vi "SetupROI.vi"(8 "error in (no error)":errorcluster, 10 "keep_first":u8) -> (0 "error out":errorcluster)   [LabVIEW 2015, in "ESLSCDLL.lvlib"]
uses:
  ESLSCDLL.lvlib
  Globals.vi
panel:
  # "if 0 every odd region is shown\nif 1 every even region is shown"
  # "number of regions 2...8"
  # "lines in camera"
  # "number of lines for each region.\nWhen selection 0 for the first region,\nthe lines are equally distributed over all regions.\nThe sum of all regions should equal lines."
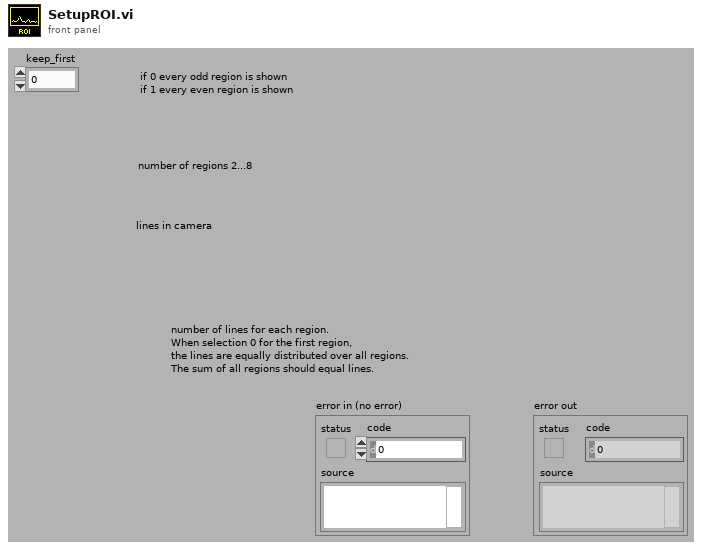
[diagram p1: front panel]
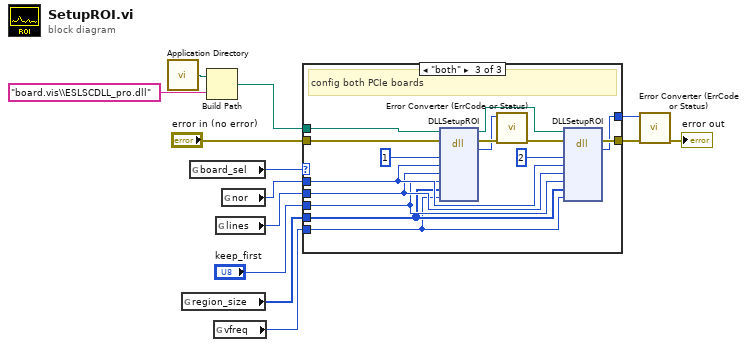
[diagram p0: block diagram]
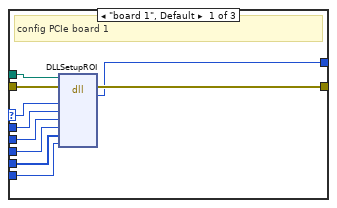
[diagram p2: hidden frame]
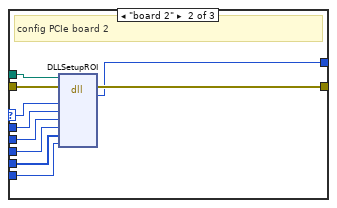
[diagram p3: hidden frame]
diagram:
  n1 = call <vilib>:"Application Directory.vi"() -> ("Application Directory"=w3:path)
  n2 = global read "Globals.vi" "region_size"() -> (w8:u32[])
  n3 = global read "Globals.vi" "board_sel"() -> (w7:enum32{"0", "board 1", "board 2", "both"})
  n4 = Build Path(base path=w3, name or relative path="board.vis\\ESLSCDLL_pro.dll") -> (appended path=w1:path)
  n5 = global read "Globals.vi" "vfreq"() -> (w4:u32)
  n6 = global read "Globals.vi" "lines"() -> (w5:u32)
  n7 = global read "Globals.vi" "nor"() -> (w6:u32)
  n8 = case shown="\"both\"" w7 {
    selector: w7 -> [w23 w33 _]
    tunnel: w6 -> [w22 w32 w46]
    tunnel: w5 -> [w21 w31 w45]
    tunnel: "keep_first" -> [w20 w30 w44]
    tunnel: w8 -> [w19 w29 w43]
    tunnel: w4 -> [w18 w28 w42]
    tunnel: "error in (no error)" -> [w17 w25 w41]
    tunnel: [w16 w27 w37] -> w10
    tunnel: [w15 w26 w36] -> w9
    tunnel: w1 -> [w14 w24 w35]
    frame "board 1", Default {
      # "config PCIe board 1"
      n9 = dll-call lib="C:/ENTW/PCIE/LV64/board.vis/ESLSCDLL_pro.dll" fn="DLLSetupROI" ("lwlscdll.dll:DLLRsTOREG")(path in=w14, error in=w17, "drv"=w23, "number_of_regions"=w22, "lines"=w21, "keep_first"=w20, "region_size"=w19, "vfreq"=w18) -> (error out=w16:errorcluster, "es_status_codes"=w15:i32)  [unwired: 7 in, 1 out]
    }
    frame "board 2" {
      # "config PCIe board 2"
      n10 = dll-call lib="C:/ENTW/PCIE/LV64/board.vis/ESLSCDLL_pro.dll" fn="DLLSetupROI" ("lwlscdll.dll:DLLRsTOREG")(path in=w24, error in=w25, "drv"=w33, "number_of_regions"=w32, "lines"=w31, "keep_first"=w30, "region_size"=w29, "vfreq"=w28) -> (error out=w27:errorcluster, "es_status_codes"=w26:i32)  [unwired: 7 in, 1 out]
    }
    frame "both" {
      # "config both PCIe boards"
      n11 = dll-call lib="C:/ENTW/PCIE/LV64/board.vis/ESLSCDLL_pro.dll" fn="DLLSetupROI" ("lwlscdll.dll:DLLRsTOREG")(path in=w35, error in=w41, "drv"=u32 1, "number_of_regions"=w46, "lines"=w45, "keep_first"=w44, "region_size"=w43, "vfreq"=w42) -> (path out=w34:path, error out=w40:errorcluster, "es_status_codes"=w39:i32)  [unwired: 7 in]
      n12 = call "Error Converter (ErrCode or Status).vi"("error in (no error)"=w40, "error code"=w39) -> ("error out"=w38:errorcluster)  [unwired: 9 in]
      n13 = dll-call lib="C:/ENTW/PCIE/LV64/board.vis/ESLSCDLL_pro.dll" fn="DLLSetupROI" ("lwlscdll.dll:DLLRsTOREG")(path in=w34, error in=w38, "drv"=u32 2, "number_of_regions"=w46, "lines"=w45, "keep_first"=w44, "region_size"=w43, "vfreq"=w42) -> (error out=w37:errorcluster, "es_status_codes"=w36:i32)  [unwired: 7 in, 1 out]
    }
  }
  n14 = call "Error Converter (ErrCode or Status).vi"("error in (no error)"=w10, "error code"=w9) -> ("error out"=→"error out":errorcluster)  [unwired: 9 in]
